vi "Reanimate.vi"(8 "Error In":errorcluster) -> (0 "Error Out":errorcluster)   [LabVIEW 2017, in "Tests.lvlib"]
uses:
  Tests.lvlib
  Support/Reanimate Target.vi
  src/Toolkit VIs/Toolkit.lvlib
  <vilib>/addons/_JKI Toolkits/Caraya/classes/Assert/Assert.lvclass
  <vilib>/addons/_JKI Toolkits/Caraya/classes/Test/Test.lvclass
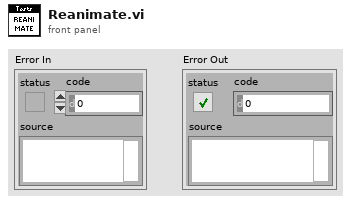
[diagram p1: front panel]
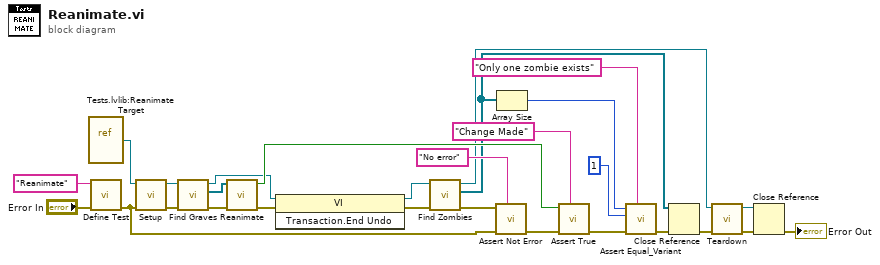
[diagram p0: block diagram]
diagram:
  n1 = vi-ref "Tests.lvlib:Reanimate Target.vi"() -> (w15:refnum<vi>)
  n2 = call <vilib>:"Define Test.vi"("error in (no error)"="Error In", "Label (VI Title)"="Reanimate") -> ("error out"=w6:errorcluster)  [unwired: 9 in]
  n3 = call "Setup.vi"("Error In"=w6, "VI In"=w15) -> ("Error Out"=w5:errorcluster, "VI Out"=w7:refnum<vi>)  [unwired: 8 in]
  n4 = call "Find Graves.vi"("Error In"=w5, "VI In"=w7) -> ("Error Out"=w11:errorcluster, "Graves"=w9:refnum<vi>[], "VI Out"=w10:refnum<vi>)  [unwired: 7 in]
  n5 = call "Reanimate.vi"("Error In"=w11, "Graves"=w9) -> ("Error Out"=w28:errorcluster, "Change Made?"=w13:bool)  [unwired: 8 in]
  n6 = invoke class="VI" method="Transaction.End Undo"(reference=w10, error in=w28) -> (reference out=w26:refnum<vi>, error out=w27:errorcluster)  [unwired: 1 in, 1 out]
  n7 = call "Find Zombies.vi"("Error In"=w27, "VI In"=w26) -> ("Error Out"=w21:errorcluster, "Graves"=w8:refnum<vi>[], "VI Out"=w2:refnum<vi>)  [unwired: 7 in]
  n8 = call <vilib>:"Assert Not Error.vi"("Label"="No error", "error in (no error)"=w6, "Not Error?"=w21) -> ("error out"=w23:errorcluster)  [unwired: 8 in]
  n9 = Array Size(array=w8) -> (size(s)=w20:i32)
  n10 = call <vilib>:"Assert True.vi"("Label"="Change Made", "error in (no error)"=w23, "True?"=w13) -> ("error out"=w14:errorcluster)  [unwired: 8 in]
  n11 = call <vilib>:"Assert Equal_Variant.vi"("Label"="Only one zombie exists", "error in (no error)"=w14, "Y"=1 ("size(s)"), "X"=w20) -> ("error out"=w17:errorcluster)  [unwired: 7 in]
  n12 = Close Reference(reference=w8, error in (no error)=w17) -> (error out=w4:errorcluster)
  n13 = call "Teardown.vi"("Error In"=w4, "VI In"=w2) -> ("Error Out"=w3:errorcluster, "VI Out"=w1:refnum<vi>)  [unwired: 8 in]
  n14 = Close Reference(reference=w1, error in (no error)=w3) -> (error out=→"Error Out":errorcluster)
